vi "Config_CheckHardware.vi"(5 "Status Ref":refnum<vi>, 6 "Ref Cluster":T1, 8 "error in (no error)":errorcluster, 10 "Config Cluster":T2={"General"={"Config.ini"=path "", "Default Logging Path"=path ""}, "Hardware"={"Global T VAR"="", "Global B VAR"="", "VISAS"={"GEN COM"="", "SCOPE COM"="", "VNA COM"=""}, "Connected?"={"SCOPE"=FALSE, "GEN"=FALSE, "VNA"=FALSE}}, "Operation"={"Operation Mode"=enum."Idle-Off", "Status"="", "NewLog?"=FALSE, "OvenWarn"=FALSE, "Scope Settings"={"TimeBase"=0.0, "VerticalScale"=4.0, "Channel"=enum."Channel 2"}, "Gen Settings"={"Amplitude"=0.0, "Frequency"=0.0, "Offset"=0.0}}}) -> (0 "error out":errorcluster, 1 "Connected?":bool, 2 "Config Cluster Out":T2={"General"={"Config.ini"=path "", "Default Logging Path"=path ""}, "Hardware"={"Global T VAR"="", "Global B VAR"="", "VISAS"={"GEN COM"="", "SCOPE COM"="", "VNA COM"=""}, "Connected?"={"SCOPE"=FALSE, "GEN"=FALSE, "VNA"=FALSE}}, "Operation"={"Operation Mode"=enum."Idle-Off", "Status"="", "NewLog?"=FALSE, "OvenWarn"=FALSE, "Scope Settings"={"TimeBase"=0.0, "VerticalScale"=4.0, "Channel"=enum."Channel 2"}, "Gen Settings"={"Amplitude"=0.0, "Frequency"=0.0, "Offset"=0.0}}})   [LabVIEW 2021]
uses:
  Config_Cluster.ctl
  Mode_Enum.ctl
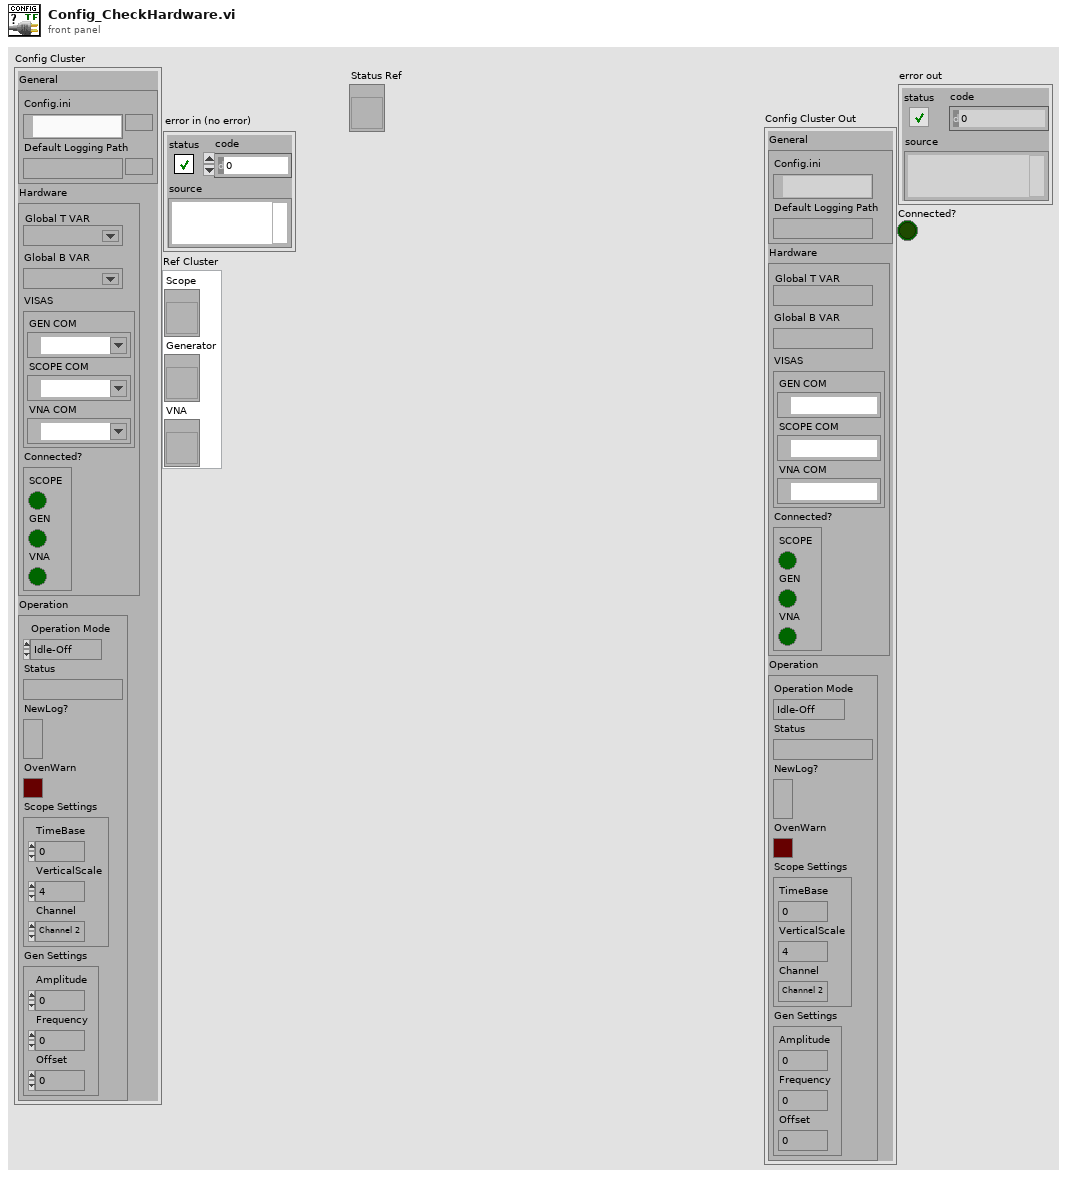
[diagram p1: front panel]
types:
  T1 = cluster{"Scope":refnum<vi>, "Generator":refnum<vi>, "VNA":refnum<vi>}
  T2 = typedef "Config_Cluster.ctl" = cluster{"General":cluster{"Config.ini":path, "Default Logging Path":path}, "Hardware":cluster{"Global T VAR":refnum<k21>, "Global B VAR":refnum<k21>, "VISAS":cluster{"GEN COM":refnum<visa-resource-name>, "SCOPE COM":refnum<visa-resource-name>, "VNA COM":refnum<visa-resource-name>}, "Connected?":cluster{"SCOPE":bool, "GEN":bool, "VNA":bool}}, "Operation":cluster{"Operation Mode":T3, "Status":string, "NewLog?":bool, "OvenWarn":bool, "Scope Settings":cluster{"TimeBase":dbl, "VerticalScale":dbl, "Channel":enum16{"Channel 2", "Channel 1"}}, "Gen Settings":cluster{"Amplitude":dbl, "Frequency":dbl, "Offset":dbl}}}
  T3 = typedef "Mode_Enum.ctl" = enum16{"Logging", "Idle-Off", "Idle"}
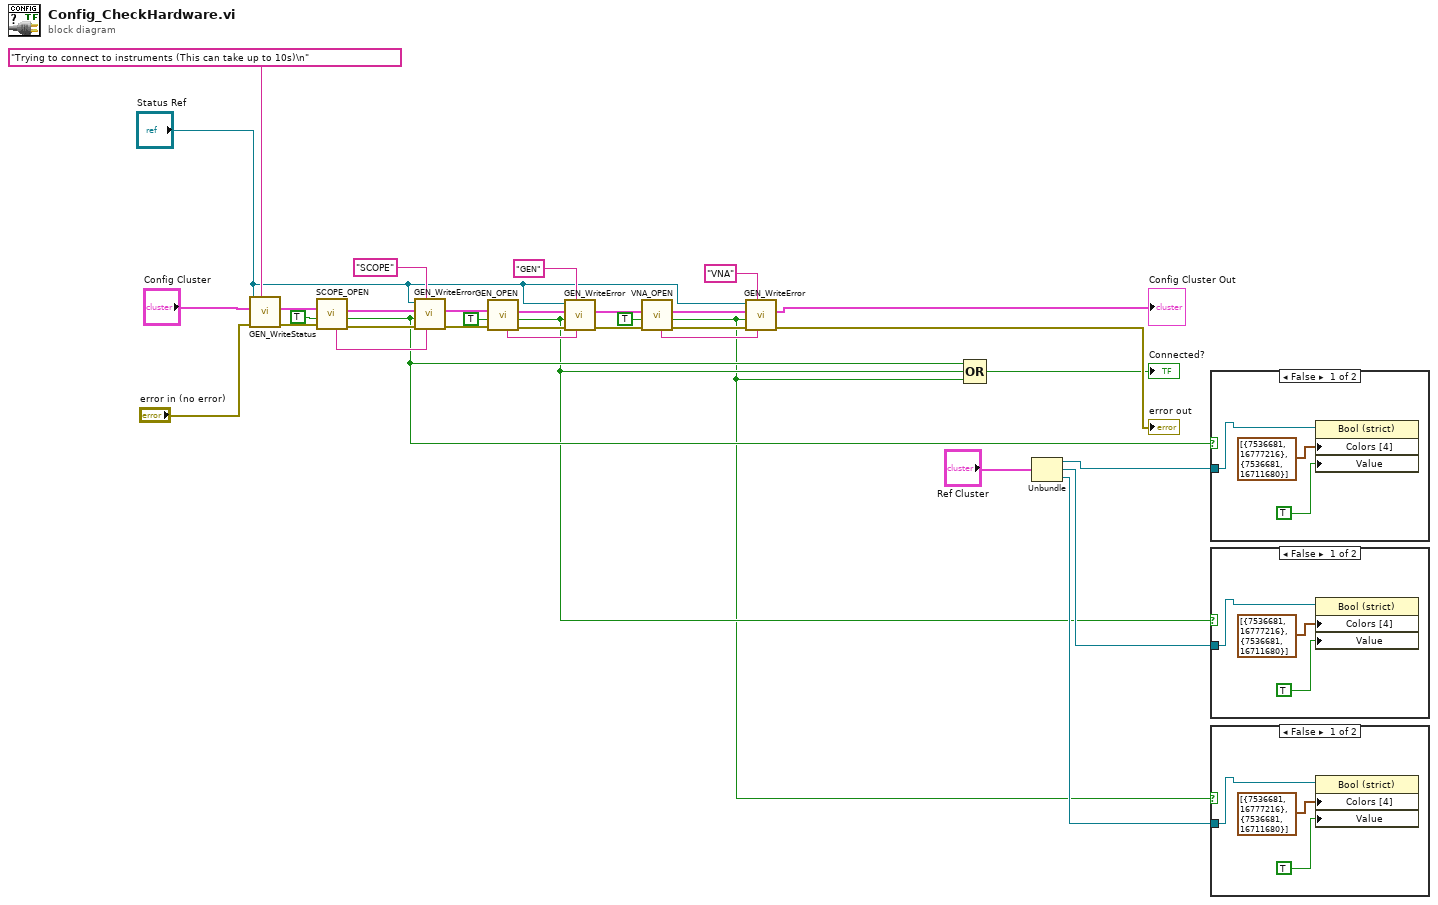
[diagram p0: block diagram]
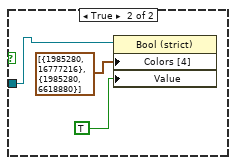
[diagram p2: hidden frame]
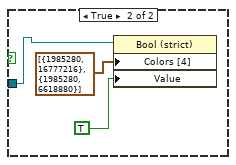
[diagram p3: hidden frame]
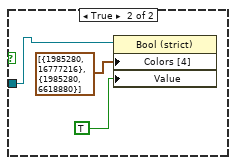
[diagram p4: hidden frame]
diagram:
  n1 = call "GEN_WriteStatus.vi"("Input String"="Trying to connect to instruments (This can take up to 10s)\n", "error in (no error)"="error in (no error)", "Config_Cluster"="Config Cluster", "Status Ref"="Status Ref") -> ("error out"=w31:errorcluster, "Config_Cluster Out"=w32:T2)  [unwired: 6 in]
  n2 = call "SCOPE_OPEN.vi"("error in (no error)"=w31, "Clear Error w/ Report?"=TRUE, "Configuration Cluster"=w32) -> ("error out"=w23:errorcluster, "Success?"=w3:bool, "Configuration Cluster Out"=w22:T2, "message"=w24:string)  [unwired: 5 in]
  n3 = call "GEN_WriteError.vi"("Error MSG"=w24, "Name"="SCOPE", "error In"=w23, "Success?"=w3, "Configuration Cluster In"=w22, "Status Ref"="Status Ref") -> ("error out"=w20:errorcluster, "Config_Cluster Out"=w21:T2)  [unwired: 4 in]
  n4 = call "GEN_OPEN.vi"("error in (no error)"=w20, "Clear Error w/ Report?"=TRUE, "Configuration Cluster"=w21) -> ("error out"=w17:errorcluster, "Success?"=w2:bool, "Configuration Cluster Out"=w18:T2, "message"=w16:string)  [unwired: 5 in]
  n5 = call "GEN_WriteError.vi"("Error MSG"=w16, "Name"="GEN", "error In"=w17, "Success?"=w2, "Configuration Cluster In"=w18, "Status Ref"="Status Ref") -> ("error out"=w13:errorcluster, "Config_Cluster Out"=w14:T2)  [unwired: 4 in]
  n6 = call "VNA_OPEN.vi"("error in (no error)"=w13, "Clear Error w/ Report?"=TRUE, "Configuration Cluster"=w14) -> ("error out"=w9:errorcluster, "Success?"=w1:bool, "Configuration Cluster Out"=w10:T2, "message"=w11:string)  [unwired: 5 in]
  n7 = call "GEN_WriteError.vi"("Error MSG"=w11, "Name"="VNA", "error In"=w9, "Success?"=w1, "Configuration Cluster In"=w10, "Status Ref"="Status Ref") -> ("error out"=→"error out":errorcluster, "Config_Cluster Out"=→"Config Cluster Out":T2)  [unwired: 4 in]
  n8 = Compound Arithmetic op=OR(w3, w2, w1) -> (→"Connected?":bool)
  n9 = Unbundle("Ref Cluster") -> ("Scope"=w29:refnum<vi>, "Generator"=w28:refnum<vi>, "VNA"=w27:refnum<vi>)
  n10 = case shown="False" w3 {
    tunnel: w29 -> [w36 w39]
    frame False {
      n11 = property class="Bool (strict)"(reference=w36, "Colors [4]"=cluster{u32, u32}[] [{7536681, 16777216}, {7536681, 16711680}], "Value"=TRUE) -> ()  [unwired: 1 in, 2 out]
    }
    frame True {
      n12 = property class="Bool (strict)"(reference=w39, "Colors [4]"=cluster{u32, u32}[] [{1985280, 16777216}, {1985280, 6618880}], "Value"=TRUE) -> ()  [unwired: 1 in, 2 out]
    }
  }
  n13 = case shown="False" w2 {
    tunnel: w28 -> [w42 w45]
    frame False {
      n14 = property class="Bool (strict)"(reference=w42, "Colors [4]"=cluster{u32, u32}[] [{7536681, 16777216}, {7536681, 16711680}], "Value"=TRUE) -> ()  [unwired: 1 in, 2 out]
    }
    frame True {
      n15 = property class="Bool (strict)"(reference=w45, "Colors [4]"=cluster{u32, u32}[] [{1985280, 16777216}, {1985280, 6618880}], "Value"=TRUE) -> ()  [unwired: 1 in, 2 out]
    }
  }
  n16 = case shown="False" w1 {
    tunnel: w27 -> [w48 w51]
    frame False {
      n17 = property class="Bool (strict)"(reference=w48, "Colors [4]"=cluster{u32, u32}[] [{7536681, 16777216}, {7536681, 16711680}], "Value"=TRUE) -> ()  [unwired: 1 in, 2 out]
    }
    frame True {
      n18 = property class="Bool (strict)"(reference=w51, "Colors [4]"=cluster{u32, u32}[] [{1985280, 16777216}, {1985280, 6618880}], "Value"=TRUE) -> ()  [unwired: 1 in, 2 out]
    }
  }
